vi "Day 2 (Part One).vi"() -> ()   [LabVIEW 2021]
panel:
  out "Score":i32
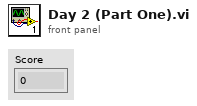
[diagram p1: front panel]
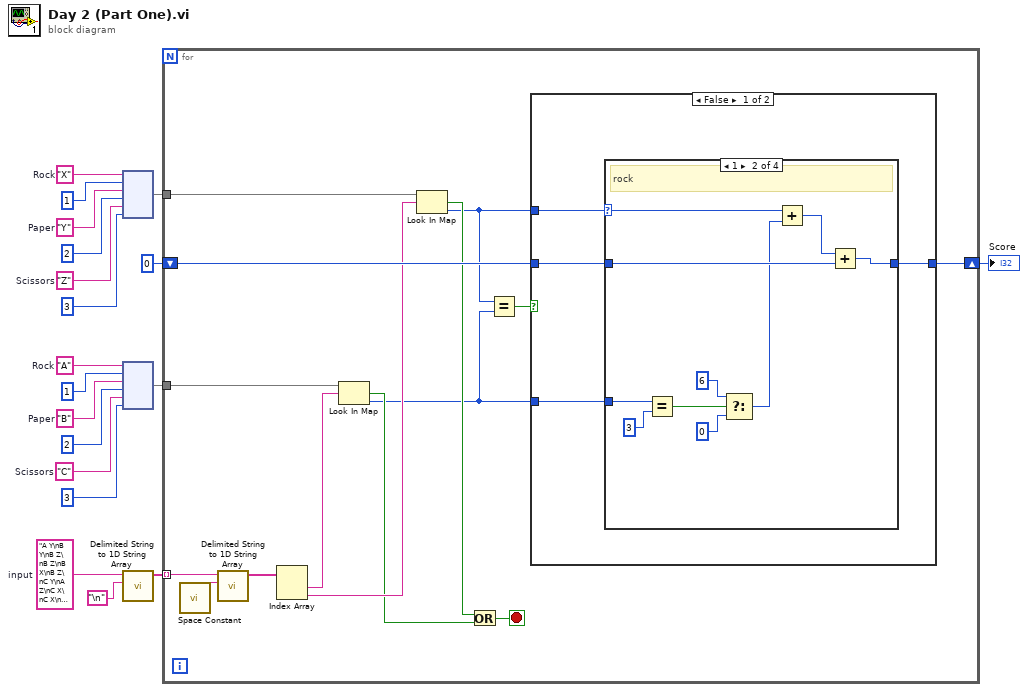
[diagram p0: block diagram]
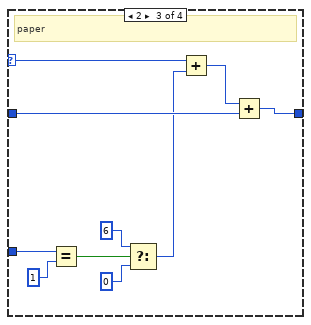
[diagram p3: hidden frame]
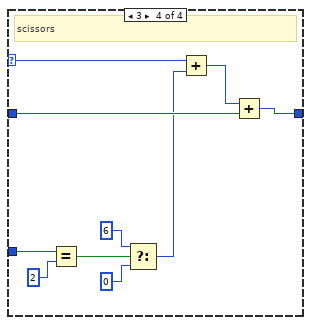
[diagram p4: hidden frame]
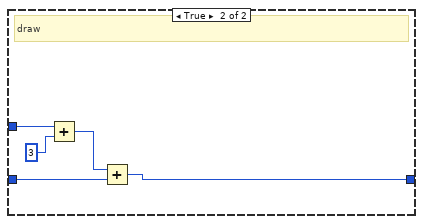
[diagram p5: hidden frame]
diagram:
  w1 = "A Y\nB Y\nB Z\nB Z\nB X\nB Z\nC Y\nA Z\nC X\nC X\nB Z\nB Z\nB Z\nA X\nB Z\nB Z\nA Y\nB Z\nA Z\nB X\nB Z\nA X\nA X\nB Z\nA Y\nA Z\nB Z\nA Y\nA Z\nB Z\nA Z\nB Z\nB Z\nC Y\nB Z\nB Z\nA X\nC X\nB Z\nA X\nB Z\nC X\nA X\nB Z\nA X\nA X\nC X\nB Z\nB Z\nB Z\nC Y\nC Y\nA X\nB Z\nC X\nB Z\nA X\nA Y\nB Z\nB Z\nB Z\nB Z\nB Z\nB X\nB Z\nB Z\nB Z\nB X\nA X\nA X\nB Z\nA Y\nC Y\nC Y\nA Y\nA X\nB Z\nA Y\nA Z\nA X\nA X\nA Y\nC Y\nB Z\nB Z\nC X\nB Z\nA Y\nA X\nB Z\nB Z\nA X\nA X\nA X\nB Z\nA Y\nB Z\nA Z\nC Y\nB Z\nB Z\nB Z\nC Y\nA Y\nC Y\nB Z\nA X\nB Z\nA X\nB Z\nC Y\nB Z\nB Z\nB Z\nC X\nB Z\nA X\nB Z\nB Z\nB Z\nA X\nA X\nB X\nC Y\nB Z\nB Z\nB Z\nA X\nB Z\nA X\nB Z\nA X\nA Z\nA X\nB Z\nA X\nC Y\nA X\nB Z\nA X\nC Y\nB Z\nB Z\nA X\nA X\nB Z\nC Y\nB Y\nB Z\nB Z\nB Z\nB X\nB Z\nB Z\nB Z\nA X\nB Z\nC Y\nC Y\nA Z\nA X\nB Z\nB Z\nB Y\nB Z\nB Z\nC Y\nB Z\nB Y\nB Z\nC Y\nB Z\nB Z\nC X\nC X\nC X\nB Z\nA Z\nA X\nC Y\nA Z\nB Z\nB Z\nB Z\nB Z\nA X\nA X\nB Z\nB Z\nA Z\nA X\nA X\nB Z\nC Y\nA X\nA Z\nA Y\nA Y\nA X\nB Z\nA X\nA Z\nB Z\nC X\nB Z\nC X\nC Y\nB Z\nB Z\nB Z\nB Z\nB Z\nC Y\nA X\nC Y\nA X\nB Y\nB Y\nA X\nA X\nB Z\nB Z\nC X\nA Z\nC Y\nA X\nA X\nA Y\nA X\nA X\nB Z\nA Z\nB Z\nB Z\nB Z\nA Z\nA X\nB Z\nB Z\nC Y\nB Z\nB Z\nB Z\nA X\nA X\nB Z\nB Z\nB Z\nB Z\nB Z\nB Z\nA X\nC X\nA X\nA X\nC Y\nA X\nB Z\nC Y\nB Z\nB Z\nB Z\nA X\nB Z\nC Y\nB Z\nA X\nA X\nB Z\nA X\nA X\nB Z\nA Z\nB X\nA X\nA X\nB Z\nC Y\nA Y\nA X\nC X\nB Z\nA X\nB Z\nB Z\nA X\nB Z\nA Z\nC Y\nB Z\nB Z\nA X\nA X\nB X\nA X\nB Z\nB Z\nC X\nA X\nC X\nA X\nB Z\nB Z\nA X\nA Z\nB Z\nB X\nA X\nA Y\nB Z\nB Z\nB Z\nC X\nC Y\nB Z\nB Z\nC Z\nB X\nC Y\nC Z\nB Z\nB Z\nA X\nB Z\nC X\nB Z\nB Z\nA Z\nA X\nC X\nB Z\nB Z\nA X\nC Y\nA X\nB X\nC Z\nB Z\nB Z\nA X\nB Z\nA Y\nB Z\nB Z\nA X\nB Z\nC Y\nC Y\nA X\nC Y\nC X\nC X\nA X\nB Z\nC Y\nB Z\nC X\nB Z\nA Z\nB Z\nA Z\nB X\nB Z\nA Z\nA X\nB Z\nB Z\nB Z\nA X\nA X\nA X\nB Z\nA X\nB Z\nB X\nA Y\nB Z\nA X\nB Z\nB Z\nB Z\nA X\nB Z\nC X\nA Y\nA X\nA Z\nC Y\nC Y\nA X\nC Y\nB Z\nA X\nB Z\nC Y\nB X\nA Z\nB Z\nB Z\nB X\nB Z\nB Z\nB Z\nA Y\nA Y\nC Y\nA Z\nA X\nB Z\nB Z\nA X\nA X\nA X\nB Z\nA X\nB Z\nB Y\nA X\nA X\nA X\nB Z\nB Z\nB Z\nC Y\nA X\nA X\nA X\nA X\nA X\nA X\nC Y\nA Z\nC X\nB Z\nB Z\nC Z\nA X\nA X\nB Z\nA X\nB X\nB Z\nB Z\nC X\nB Z\nA Z\nA X\nB Z\nA Z\nB Z\nB Y\nA X\nC Y\nA X\nB Z\nB Z\nB Z\nA Z\nC Y\nC Z\nA X\nB Z\nB Z\nB X\nA X\nB Z\nA X\nB Z\nB Z\nC Z\nB Z\nA X\nC Y\nC X\nA Z\nC X\nA X\nA X\nA X\nB Z\nB Y\nC Y\nB Z\nB Z\nC Y\nB Z\nA X\nB Z\nA Z\nA X\nB Z\nA Y\nA X\nA X\nB X\nB Z\nB Z\nB Z\nB Z\nC Z\nB Y\nA X\nA X\nB Z\nB Z\nB Z\nC Z\nB Z\nB Z\nA Y\nA Z\nB Z\nA X\nC Y\nB Z\nA Z\nC Z\nB Z\nC X\nB Z\nB Z\nA X\nB Z\nA X\nB Z\nC Y\nA X\nB Z\nA Z\nB Z\nC Y\nA X\nC X\nA X\nA X\nB Z\nB Z\nB X\nB Z\nC X\nC Y\nA Z\nB Z\nC Y\nB Z\nC Y\nB Y\nA Y\nB Z\nA X\nB Z\nA Z\nB Z\nA X\nC X\nB Z\nB X\nC Y\nA Z\nA X\nB Z\nB Z\nB Z\nA Z\nC Y\nC Y\nB Z\nA Y\nA X\nA X\nA Y\nC Y\nA Y\nB Z\nB Z\nB Z\nA Z\nB Z\nA Z\nB Z\nA X\nA Z\nB Z\nC Y\nB Z\nA X\nA X\nA X\nA Z\nA Z\nB Z\nC Y\nB Z\nA X\nB Z\nB Z\nA Z\nB Z\nB Z\nA X\nB Z\nB Z\nB X\nA X\nB Z\nB Z\nA Z\nA X\nB X\nA X\nB Z\nA X\nB Z\nA X\nB Z\nC Y\nB Z\nC Z\nC X\nB Z\nB Z\nB Z\nC Y\nC X\nB Z\nB Z\nB Z\nB Z\nA Y\nA Y\nC Y\nA X\nC X\nB X\nA X\nC X\nA Y\nB X\nA X\nA Z\nB Z\nB X\nB Y\nB Z\nB Z\nB X\nB Z\nC Y\nB Z\nA X\nA X\nA X\nB Z\nA X\nB Z\nA X\nB Z\nB Z\nB Z\nB Z\nA X\nC Y\nA X\nB Z\nB Z\nB Z\nA X\nB Z\nB Z\nC Z\nA X\nA Z\nB Z\nC Y\nB Z\nB Z\nB Z\nB Z\nA Z\nB Z\nB Z\nB Z\nC Y\nA X\nB X\nC Y\nA X\nC Z\nB Z\nC Y\nC Y\nB Z\nA X\nB Z\nC Z\nA X\nA Z\nB Z\nA Z\nB Z\nB X\nB Z\nA Z\nB Z\nC Y\nC Z\nB Z\nA X\nB Z\nA X\nA X\nB Z\nB Z\nB Z\nB Z\nA X\nA Z\nA X\nB X\nB Z\nA Y\nA Y\nB Z\nA X\nB Z\nB Z\nA Y\nC X\nB Z\nB Z\nB Z\nC X\nB Z\nC X\nA X\nB Z\nC Y\nA X\nA X\nA X\nC Z\nA X\nA X\nA Y\nB Z\nB Z\nB Z\nB Z\nB Z\nC X\nC Y\nB Z\nB Z\nC X\nB Z\nB Z\nB Z\nC Y\nC Y\nA Z\nA X\nB Z\nA X\nB X\nB Z\nB Z\nC Y\nB Z\nA X\nB X\nA Z\nA Z\nB Z\nA X\nC X\nA X\nB Z\nB Z\nB Z\nA X\nA Z\nC X\nB Z\nA X\nA Z\nA Z\nA Z\nA Z\nC Y\nB X\nB X\nC Z\nB X\nC Z\nA X\nA Y\nB Z\nB X\nA Y\nA Z\nB X\nA X\nA X\nC Z\nA Z\nB Z\nC X\nB Z\nB Z\nC X\nB Z\nC X\nA X\nA Y\nA X\nB Z\nA X\nB Z\nC Y\nB Z\nB Z\nB Z\nB Z\nB Z\nB Z\nB Z\nB Z\nB Z\nA X\nB Z\nA X\nB Z\nA Y\nB Z\nA X\nA Z\nB Z\nC Y\nA Z\nA X\nA Z\nC X\nB Z\nB Z\nB Z\nA X\nC X\nC Y\nB Z\nA Z\nA Z\nC X\nB Z\nC Y\nA Z\nA Z\nA Y\nB Z\nA Z\nB Z\nB Y\nC Y\nB Z\nB Z\nA Z\nA X\nB Z\nC Y\nB Z\nB Z\nB Z\nB Z\nB Z\nA X\nC Y\nB X\nC X\nB Z\nA Z\nB Z\nA X\nB Z\nB Z\nA X\nC Y\nA X\nA X\nA X\nC X\nA X\nA X\nB Z\nA Y\nA X\nB Z\nC X\nA X\nC Z\nA X\nB Z\nC X\nA X\nA X\nA X\nB Z\nC X\nB Z\nB Z\nA X\nA X\nA X\nA X\nB Z\nA X\nA X\nB Z\nB X\nA Y\nA X\nC X\nA X\nC X\nA X\nB Z\nB Z\nB Z\nB Z\nB Z\nA X\nA X\nB X\nC Y\nA Y\nC X\nC X\nC X\nB Z\nB Z\nB X\nB Z\nB Z\nC X\nB Z\nB Z\nA X\nB Z\nB Z\nB X\nA X\nA X\nC Y\nC X\nA X\nC Y\nA Y\nC X\nB Z\nA X\nA Z\nB Z\nB Z\nB X\nB Z\nB Z\nB Z\nC Y\nB X\nA X\nB Z\nA X\nB Z\nA X\nA Z\nA Y\nC Y\nB Z\nC Y\nA Z\nA Z\nB Z\nA X\nA X\nC Y\nC Y\nA X\nB Z\nA X\nC X\nC Z\nA X\nA Y\nA X\nA X\nA X\nB Z\nB Z\nB Z\nC Y\nB Z\nB Z\nC Z\nA X\nB Z\nB Z\nA X\nA X\nB Z\nB Z\nB Z\nA Y\nB X\nA Z\nA Z\nB Z\nA X\nB Z\nB Y\nA Y\nA X\nC Y\nA Z\nB Z\nC X\nC X\nA X\nB Z\nA X\nA X\nA Z\nB Z\nA Z\nA Z\nB Z\nB Z\nA Y\nB Z\nC Y\nC X\nB Z\nA X\nA X\nB Z\nB Z\nA X\nA X\nC Y\nB Z\nA Z\nA X\nB Z\nC Y\nB Z\nA X\nA X\nB X\nA X\nB Z\nC Y\nB Z\nA Y\nB Z\nB Z\nB Z\nB X\nA X\nB Z\nC Y\nB Z\nB Z\nB Z\nA Z\nC Y\nC Y\nC Y\nA X\nA Z\nA X\nB Z\nA X\nB Z\nA X\nC Y\nB Z\nB Z\nA X\nB Z\nA X\nA X\nB Z\nB Z\nA X\nA X\nC X\nB Z\nA Y\nA X\nA X\nB Z\nC Y\nC X\nC X\nB Y\nA Z\nB Z\nA Z\nA X\nB Z\nC Y\nB Z\nA X\nA Z\nB Z\nA X\nA Y\nA X\nB Z\nB Z\nB Y\nB Z\nA X\nB Z\nB Z\nB Z\nC Y\nA X\nB Z\nB Z\nA X\nA X\nA X\nB Z\nA Y\nB Z\nA Z\nA X\nB Z\nC X\nB Z\nA X\nA Z\nA Z\nB Z\nA X\nB Z\nB Z\nB Z\nB Z\nC Y\nA Y\nA Z\nA X\nA Y\nB Z\nB Z\nB Z\nC Y\nC Y\nB Z\nA Y\nA Z\nA X\nB Z\nA Z\nB Z\nA X\nC Y\nB Z\nB Z\nB Z\nB Z\nB Z\nC X\nA Z\nB Z\nA Z\nB Z\nA X\nB Z\nA X\nA Y\nB Z\nB X\nB Z\nA Y\nB Z\nA Z\nB Z\nB Z\nA X\nA Z\nA Z\nB X\nB Z\nA X\nB X\nA X\nA Z\nA X\nC X\nB Z\nC X\nA X\nC X\nA X\nA X\nA Z\nA Z\nB Z\nA Z\nB X\nB Z\nB Z\nA X\nB Z\nB Z\nA X\nB Z\nB Z\nB Z\nB Z\nB Z\nC X\nA X\nC Y\nB Z\nB Z\nA Y\nB X\nB Z\nA Z\nB Z\nB Z\nC Y\nB Z\nA X\nA Z\nB Z\nA Z\nB Z\nB Z\nA X\nB Z\nA Z\nA Z\nA Z\nC X\nA Z\nB Z\nC Y\nB Z\nA Z\nB Z\nA X\nA X\nA X\nA Z\nA X\nB Z\nB Z\nB Z\nB Z\nA Y\nA X\nC Y\nC Z\nB Z\nA Z\nA X\nB Z\nB X\nB Z\nA X\nB Z\nB Z\nC Y\nA X\nB Z\nB Z\nC X\nC X\nB Z\nB Y\nA Y\nA X\nC Y\nA X\nA X\nB Z\nB Z\nB Z\nB Z\nA Z\nC X\nA X\nA X\nA X\nA X\nA Y\nA Z\nA Y\nA Y\nB Z\nA X\nA Y\nA X\nA Z\nA Z\nA X\nB Z\nB Z\nC Y\nA X\nB Z\nC Y\nB Z\nB Z\nA X\nB Z\nB X\nA X\nB Z\nA Y\nA Y\nB X\nB Z\nB Z\nC X\nA X\nB Z\nA X\nB X\nB Z\nA X\nB Z\nA X\nB X\nA X\nA X\nC X\nA X\nA X\nB Z\nA X\nA X\nA Y\nB Z\nB Z\nC Y\nB Z\nA X\nB Z\nB Z\nA Z\nA X\nB Z\nA Y\nB Z\nC Y\nA Z\nA X\nA Y\nC Y\nA X\nA Y\nC X\nB Z\nA X\nA Y\nA X\nB Z\nA Z\nB Z\nB Z\nC Y\nA X\nC Y\nA Z\nB Z\nB Z\nA X\nA X\nB X\nB Z\nC Y\nB Z\nB Y\nA X\nB Z\nA X\nC X\nB Z\nA Y\nA X\nB Z\nC Y\nA Z\nB Z\nA X\nA X\nA Y\nA Z\nC X\nB Z\nB Z\nB Z\nA Z\nB Z\nC Y\nB Z\nB Z\nB Z\nB Z\nB X\nB Z\nA X\nB Z\nB Z\nA X\nC X\nC Y\nB Z\nB Z\nA X\nB Z\nA X\nA X\nA Y\nB Z\nA Z\nB Z\nC Y\nB Z\nA X\nA Y\nC Y\nB Y\nA Y\nA X\nC Y\nA X\nA Z\nA X\nB Z\nA Z\nB Z\nA X\nB Z\nC Y\nA X\nB Z\nB X\nB Z\nA X\nA X\nA X\nB Z\nA Z\nA Z\nB Z\nA X\nB Z\nB Z\nA X\nA X\nB Z\nB Z\nA X\nB Z\nB X\nB Z\nC Y\nA Z\nB X\nA X\nB Z\nB Z\nA X\nB Z\nA X\nB Z\nB X\nB X\nA X\nB Z\nB Z\nB Z\nB Z\nA Y\nB Z\nB Z\nA X\nC X\nB Z\nB Z\nB Z\nB Z\nB Z\nA X\nC X\nA Y\nA X\nA X\nB Z\nC Y\nC X\nB Z\nA X\nA Y\nB Z\nA X\nB Z\nC Y\nB Z\nA X\nB Z\nA Y\nB X\nA X\nB Z\nA X\nB Z\nA X\nB Z\nA X\nC X\nC X\nA X\nB Z\nA Y\nB Z\nB Z\nA X\nA X\nB Z\nB Z\nB Z\nA X\nA X\nA X\nC Y\nA Y\nB Z\nB Z\nB Z\nB Z\nA X\nA X\nB Z\nB Z\nC Y\nA X\nA X\nB Z\nA X\nA Y\nA X\nB Z\nB Z\nB Z\nA X\nB Z\nA X\nB Z\nA X\nA X\nB Z\nA Y\nA Z\nB Y\nA X\nA Z\nB Z\nB Z\nA Z\nA X\nA X\nB Z\nA X\nB Z\nA X\nC X\nA Z\nA X\nB Z\nB Z\nA X\nA Z\nC X\nB Z\nB Z\nA X\nB Z\nB Z\nA X\nB Z\nB Z\nB Z\nA Y\nA Z\nB Z\nB Z\nA X\nB Z\nB Z\nB X\nC X\nB Z\nB Z\nB Z\nA X\nA X\nA Z\nB Z\nC X\nB Y\nA Y\nB Z\nB Z\nA X\nA X\nA Z\nB Z\nB Z\nB Z\nA X\nA Z\nA X\nB Z\nB Z\nA Z\nB Z\nA Y\nA Z\nC Y\nB Z\nB Z\nB Z\nB Z\nA Z\nA Z\nA Y\nB Z\nA X\nA X\nB Z\nA Z\nB Z\nB Z\nB X\nC Y\nB Z\nC Y\nB Z\nA X\nC Z\nB Z\nA X\nA X\nB Z\nA Z\nA X\nB Z\nA Z\nA X\nC Z\nC X\nB Z\nB Z\nB Z\nB Z\nB Z\nC Y\nA X\nB Z\nC Y\nA X\nB Z\nB Z\nA Z\nA Z\nB Z\nC Y\nA X\nC X\nB Z\nB Z\nB Z\nB Z\nA X\nB Z\nA X\nB Z\nA Y\nB Z\nB Z\nB Z\nB Z\nB Z\nC Y\nB Z\nB Z\nA X\nA X\nA X\nA Z\nB Z\nA Y\nC Z\nA Z\nB Z\nB Z\nB Z\nA X\nB X\nC Y\nC X\nC Y\nB Z\nB Z\nB Z\nB Z\nA Y\nB Z\nA X\nC X\nA X\nB X\nC X\nB Z\nB Z\nA X\nA X\nC Y\nC Y\nA X\nB Z\nC Y\nA Y\nA Z\nA Y\nB Z\nB Z\nB Z\nA Y\nB Z\nA Z\nA X\nB Z\nC X\nA Z\nB Z\nA X\nC X\nA X\nC Y\nB X\nB Z\nB Z\nA X\nC Y\nA X\nB Z\nC X\nA Z\nA Y\nB Z\nA Z\nB Z\nB Z\nB Z\nB Z\nA X\nA X\nB Z\nA Z\nC Y\nA Y\nA X\nA X\nB Z\nC Z\nB Z\nA Z\nB X\nC X\nB Z\nB Z\nA X\nA Z\nA X\nA Z\nA X\nB Z\nB Z\nC Y\nB Z\nB Z\nB Z\nB Z\nA Z\nB Z\nB X\nB Z\nB Z\nB Z\nB Z\nC X\nC X\nA X\nB Z\nB Z\nB Z\nB Z\nB Z\nB Z\nA X\nC X\nB Z\nB Z\nA Y\nB Z\nA X\nC Y\nB Z\nC Y\nB Z\nA Y\nB Z\nB Z\nB Z\nA X\nA X\nA X\nB Z\nC Y\nB Z\nA Z\nA Y\nA Z\nA Y\nB Z\nA X\nB X\nB Z\nA X\nB Z\nA Y\nA X\nB Z\nA X\nA X\nA Y\nA Y\nA X\nA X\nA X\nB Z\nB Z\nB Z\nA X\nB Z\nA X\nB Z\nA X\nB Y\nB Y\nA X\nB Z\nC X\nA Z\nC Y\nA X\nB Z\nB Z\nB Z\nC Y\nB X\nC Y\nB Z\nB Z\nB Z\nA Z\nB Z\nB Z\nB Z\nC Y\nB Z\nB Z\nA X\nA Z\nA Y\nC Y\nB Z\nB Z\nA X\nB Z\nB Z\nA X\nA X\nB Z\nB Y\nB Z\nB Z\nA Z\nB Z\nB Z\nA X\nB Z\nA X\nC X\nC X\nA X\nC Y\nB Z\nB Z\nB Z\nA X\nC Y\nB Z\nB Z\nB Z\nB Z\nB Z\nB Z\nB Z\nB Z\nB Z\nB Z\nC Y\nC X\nB Z\nB Z\nB Z\nC Y\nA Y\nC Y\nA X\nB X\nB Z\nA X\nC X\nB Z\nA Z\nC X\nC X\nB Z\nB Z\nA Z\nB Z\nB X\nB Z\nB Z\nB Z\nA X\nC X\nB Z\nA X\nC Y\nB Z\nB Z\nC X\nB X\nA X\nB Z\nC X\nC X\nB Z\nB X\nA X\nB Z\nA Y\nB Z\nA Z\nA X\nB Z\nA X\nA X\nB Z\nB Z\nA X\nB Z\nA X\nA X\nC Y\nB Z\nA X\nC Y\nB Z\nB Z\nA X\nA Y\nC Y\nB Z\nA X\nB Z\nA X\nA X\nB Z\nB Z\nC Y\nB Z\nA X\nA X\nA X\nA X\nA Z\nB Z\nB Z\nC X\nC X\nB Z\nB Z\nC Y\nB Z\nA Y\nB Z\nA X\nC X\nA Z\nB Z\nB Z\nB Z\nC Y\nA X\nB Z\nB Z\nC Y\nB Z\nC Y\nB Z\nA Z\nB Z\nA X\nB Z\nC Y\nC Y\nA X\nA X\nA Z\nB Z\nC Y\nC Y\nA X\nB Z\nB Z\nA X\nB Z\nB Z\nB Z\nB Z\nB X\nB Y\nA X\nB Z\nB Z\nB Z\nC Y\nA X\nA Y\nB Z\nA Z\nA Z\nB X\nA X\nC Y\nB Z\nB Z\nA Z\nB Z\nC X\nC X\nA Z\nB Z\nA X\nB Z\nA X\nB Z\nB Z\nB X\nA X\nA Z\nB X\nA X\nB Z\nA X\nA X\nA Z\nA Y\nB Z\nA Y\nC Y\nC X\nB Z\nB Z\nA X\nA X\nB Z\nB Z\nB Z\nA Z\nC X\nA X\nB Z\nB Z\nA X\nB Z\nB Z\nB Z\nA X\nA Z\nB Z\nA X\nB Z\nA X\nB Z\nB Z\nA X\nC Y\nA X\nC X\nA Z\nB X\nA Y\nA Y\nB Z\nB Z\nB Z\nA X\nA X\nA X\nA Y\nB Z\nB Z\nB Z\nB Z\nB Z\nB Z\nB Z\nB Z\nC Y\nB Z\nB Z\nB Z\nC Y\nA X\nA Z\nB Z\nC Y\nB Z\nA Z\nA X\nB Z\nA Y\nB Z\nB Z\nA Z\nB Z\nA X\nA Z\nA Z\nB Z\nB Z\nB Z\nB Z\nA X\nA Z\nB Z\nB Z\nB Z\nB Z\nA Z\nB Z\nC X\nB Z\nB Y\nA X\nB Z\nB Z\nA X\nB Z\nA X\nA X\nA X\nA X\nB X\nB Z\nC X\nB Z\nB Z\nB Z\nA X\nB Z\nC X\nB Z\nA Z\nA X\nA X\nB Z\nB Z\nB Z\nB Z\nC X\nA X\nB Z\nB Z\nC Y\nB Z\nC Y\nB Z\nB Z\nA X\nB Z\nA X\nA Y\nB Z\nA Z\nB Z\nB Z\nA Y\nB Z\nB Z\nC Y\nA X\nA X\nA X\nA X\nB Z\nB Z\nA Y\nB Z\nA Z\nA X\nA X\nB Z\nA Y\nB Z\nB Z\nB X\nA Y\nA X\nA X\nC Y\nC X\nA X\nB Z\nB Z\nB Z\nA Y\nB Z\nC X\nC X\nC X\nB Z\nB Z\nB Z\nB Z\nB Z\nA X\nB Z\nA Y\nB Z\nA Y\nC X\nB X\nB Z\nB Z\nA X\nB X\nB Z\nB Z\nB Z\nB Z\nB Z\nA X\nB Z\nC X\nB X\nA X\nA X\nA X\nA X\nA X\nB Z\nC X\nC Y\nA X\nB Z\nC X\nA Z\nB Z\nB Z\nC Y\nA X\nA Z\nB Z\nB Z\nB Z\nB Z\nB Z\nB Z\nA X\nA X\nB X\nA X\nB Z\nA X\nB Z\nB Z\nA Z\nB Z\nB Z\nB Z\nB Z\nC X\nB Z\nA Z\nB Z\nB Z\nA Z\nA X\nC X\nB X\nC X\nA X\nB Z\nA Z\nB X\nB X\nA Z\nB Z\nB Z\nB X\nB Z\nB Z\nC X\nA Y\nA X\nA Z\nB Z\nA X\nB Z\nB Z\nB Z\nB Z\nA X\nA X\nC Y\nB Z\nB Z\nB Z\nA Z\nC X\nC Y\nB Y\nB Z\nB Z\nA X\nC Y\nA Z\nB Z\nB Z\nB Z\nB Z\nB Z\nC X\nB Z\nA X\nC X\nA X\nA Z\nC Y\nC X\nB Z\nB Z\nA Y\nA Z\nA Z\nA X\nA Z\nA Z\nC Y\nB Z\nB Z\nB Z\nB Z\nA Z\nA X\nA Y\nC X\nA X\nB Z\nB Z\nB Z\nA X\nB Z\nB Z\nA Z\nB Z\nA X\nB Z\nA X\nA Y\nB Z\nA X\nA Z\nB Z\nA X\nB Z\nC X\nB Z\nB Z\nC X\nA Y\nB Z\nA Z\nC X\nC Z\nC X\nB Z\nB Z\nB Z\nA X\nB Z\nC X\nA X\nA Y\nA X\nA Z\nC Y\nA X\nB Z\nB Z\nC Z\nA X\nB Z\nB Z\nA X\nA Z\nB Z\nA Y\nB Z\nC X\nA X\nA X\nB Z\nB Z\nB Z\nB X\nC X\nB Z\nB Z\nA X\nA X\nA Z\nB Z\nB Z\nA Z\nC Y\nC Z\nB Z\nA X\nA X\nA X\nC Y\nA X\nA X\nA X\nA Z\nB Z\nA Y\nB Z\nC X\nB Z\nA X\nC X\nB Z\nA Y\nA X\nB Z\nB Z\nB Z\nA X\nA Y\nB Z\nA X\nB Z\nB Z\nB Z\nB Z\nA X\nA X\nB Z\nC X\nB X\nA Z\nB Z\nB Z\nB Z\nB Z\nB Z"  # input
  w9 = "Z"  # Scissors
  w11 = "Y"  # Paper
  w6 = "X"  # Rock
  w14 = "C"  # Scissors
  w12 = "B"  # Paper
  w17 = "A"  # Rock
  n1 = node(w6, 1 ("value"), w11, 2 ("value"), w9, 3 ("value")) -> (w4:map{string, i32})
  n2 = node(w17, 1 ("value"), w12, 2 ("value"), w14, 3 ("value")) -> (w5:map{string, i32})
  n3 = call <vilib>:"Delimited String to 1D String Array.vi"("delimiter"="\n", "delimited string"=w1) -> ("string array"=w18:string[])  [unwired: 9 in]
  n4 = for {
    tunnel: w18 -> [w34] mode=indexing
    tunnel: w4 -> [w32]
    tunnel: w5 -> [w31]
    shift-right: [w29] -> w2
    shift-left: 0 -> [w30]
    stop <- w22 stop-if-true
    n5 = call <vilib>:"Space Constant.vi"() -> ("String"=w33:string)
    n6 = call <vilib>:"Delimited String to 1D String Array.vi"("delimiter"=w33, "delimited string"=w34) -> ("string array"=w27:string[])  [unwired: 9 in]
    n7 = Index Array(array=w27) -> (element #1=w25:string, element #2=w26:string)  [unwired: 2 in]
    n8 = Look In Map(map=w31, key=w25) -> (key not found?=w24:bool, value=w20:i32)  [unwired: 1 in]
    n9 = Look In Map(map=w32, key=w26) -> (key not found?=w23:bool, value=w21:i32)  [unwired: 1 in]
    n10 = Or(x=w23, y=w24) -> (x .or. y?=w22:bool)
    n11 = Equal?(x=w21, y=w20) -> (x = y?=w28:bool)
    n12 = case shown="False" w28 {
      tunnel: w21 -> [w35 w74]
      tunnel: w20 -> [w37 _]
      tunnel: w30 -> [w38 w72]
      tunnel: [w36 w71] -> w29
      frame False {
        n13 = case shown="1" w35 {
          selector: w35 -> [_ w43 w53 w63]
          tunnel: w38 -> [w39 w49 w59 w69]
          tunnel: w37 -> [_ w46 w56 w66]
          tunnel: [w39 w48 w58 w68] -> w36
          frame Default {
          }
          frame 1 {
            # "rock"
            n14 = Equal?(x=w46, y=3) -> (x = y?=w44:bool)
            n15 = Select(t=6, s=w44, f=0) -> (s? t:f=w42:i32)
            n16 = Add(x=w43, y=w42) -> (x+y=w47:i32)
            n17 = Add(x=w47, y=w49) -> (x+y=w48:i32)
          }
          frame 2 {
            # "paper"
            n18 = Equal?(x=w56, y=1) -> (x = y?=w54:bool)
            n19 = Select(t=6, s=w54, f=0) -> (s? t:f=w52:i32)
            n20 = Add(x=w53, y=w52) -> (x+y=w57:i32)
            n21 = Add(x=w57, y=w59) -> (x+y=w58:i32)
          }
          frame 3 {
            # "scissors"
            n22 = Equal?(x=w66, y=2) -> (x = y?=w64:bool)
            n23 = Select(t=6, s=w64, f=0) -> (s? t:f=w62:i32)
            n24 = Add(x=w63, y=w62) -> (x+y=w67:i32)
            n25 = Add(x=w67, y=w69) -> (x+y=w68:i32)
          }
        }
      }
      frame True {
        # "draw"
        n26 = Add(x=w74, y=3) -> (x+y=w70:i32)
        n27 = Add(x=w70, y=w72) -> (x+y=w71:i32)
      }
    }
  }
  "Score" <- w2
